vi "SubSystems.vi"(8 "error in":errorcluster) -> ()   [LabVIEW 2018]
doc: "This VI calls the various robot subsystems that will then run in parallel. New subSystems will automatlically script code to make the call."
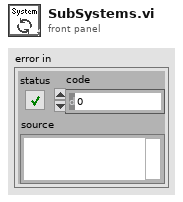
[diagram p1: front panel]
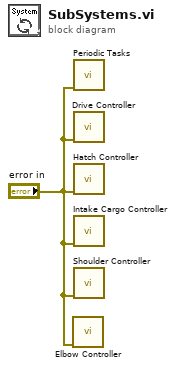
[diagram p0: block diagram]
diagram:
  n1 = call "Elbow Controller.vi"("error in"="error in") -> ()  [unwired: 11 in]
  n2 = call "Periodic Tasks.vi"("error in"="error in") -> ()  [unwired: 1 in, 10 out]
  n3 = call "Drive Controller.vi"("error in"="error in") -> ()  [unwired: 11 in]
  n4 = call "Hatch Controller.vi"("error in"="error in") -> ()  [unwired: 11 in]
  n5 = call "Intake Cargo Controller.vi"("error in"="error in") -> ()  [unwired: 11 in]
  n6 = call "Shoulder Controller.vi"("error in"="error in") -> ()  [unwired: 11 in]
